vi "blok_danych(SubVI).vi"(6 "samples":i32=128, 7 "liczba cykli":i64, 9 "Amp":dbl, 10 "phase":dbl, 11 "Sygnal":T1(ring)) -> (3 "Gaussian noise pattern":dbl[](array[numeric]))   [LabVIEW 2025]
uses:
  <vilib>/Analysis/NI_AALBase.lvlib
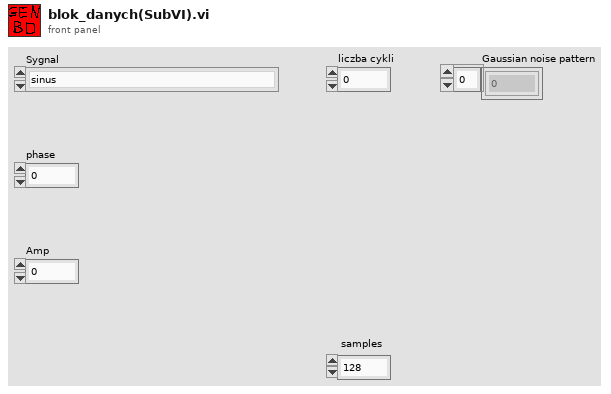
[diagram p1: front panel]
types:
  T1 = enum16{"sinus", "prostokat", "pila", "trojkat", "rozklad losowy", "rozklad normalny"}
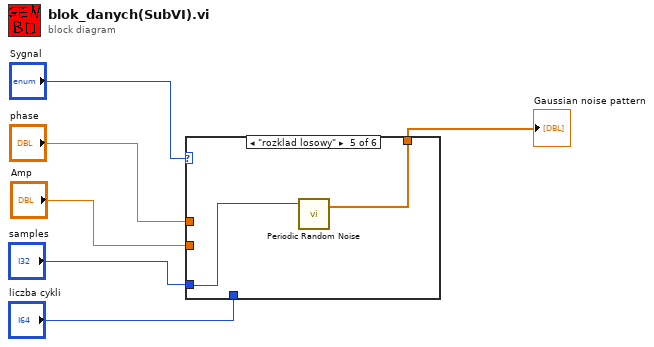
[diagram p0: block diagram]
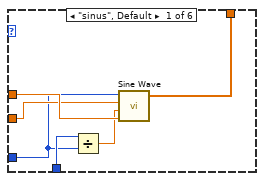
[diagram p2: hidden frame]
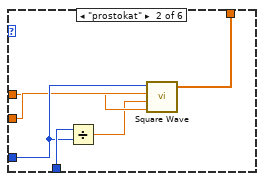
[diagram p3: hidden frame]
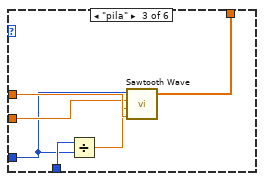
[diagram p4: hidden frame]
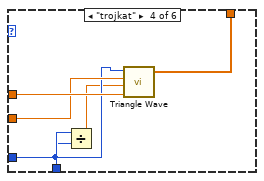
[diagram p5: hidden frame]
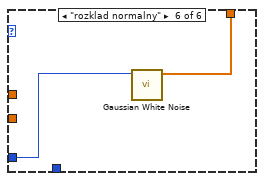
[diagram p6: hidden frame]
diagram:
  n1 = case shown="\"rozklad losowy\"" "Sygnal" {
    tunnel: "phase" -> [w12 w15 w24 w30 _ _]
    tunnel: "Amp" -> [w11 w16 w23 w29 _ _]
    tunnel: [w7 w13 w19 w28 w31 w33] -> w4
    tunnel: "samples" -> [w9 w17 w21 w26 w32 w34]
    tunnel: "liczba cykli" -> [w10 w18 w22 w27 _ _]
    frame "sinus", Default {
      n2 = Divide(x=w10, y=w9) -> (x/y=w8:dbl)
      n3 = call <vilib>:"Sine Wave.vi"("samples"=w9, "amplitude"=w11, "frequency"=w8, "phase in"=w12) -> ("sine wave"=w7:dbl[])  [unwired: 1 in, 2 out]
    }
    frame "prostokat" {
      n4 = Divide(x=w18, y=w17) -> (x/y=w14:dbl)
      n5 = call <vilib>:"Square Wave.vi"("samples"=w17, "amplitude"=w16, "frequency"=w14, "phase in"=w15) -> ("square wave"=w13:dbl[])  [unwired: 2 in, 2 out]
    }
    frame "pila" {
      n6 = Divide(x=w22, y=w21) -> (x/y=w20:dbl)
      n7 = call <vilib>:"Sawtooth Wave.vi"("samples"=w21, "amplitude"=w23, "frequency"=w20, "phase in"=w24) -> ("sawtooth wave"=w19:dbl[])  [unwired: 1 in, 2 out]
    }
    frame "trojkat" {
      n8 = Divide(x=w27, y=w26) -> (x/y=w25:dbl)
      n9 = call <vilib>:"Triangle Wave.vi"("samples"=w26, "amplitude"=w29, "frequency"=w25, "phase in"=w30) -> ("triangle wave"=w28:dbl[])  [unwired: 1 in, 2 out]
    }
    frame "rozklad losowy" {
      n10 = call <vilib>:"Periodic Random Noise.vi"("samples"=w32) -> ("periodic random noise"=w31:dbl[])  [unwired: 2 in, 1 out]
    }
    frame "rozklad normalny" {
      n11 = call <vilib>:"Gaussian White Noise.vi"("samples"=w34) -> ("Gaussian noise pattern"=w33:dbl[])  [unwired: 9 in, 1 out]
    }
  }
  "Gaussian noise pattern" <- w4
